vi "Stop.vi"(0 "object in":refnum<class "CetoniPump.lvclass">, 2 "index":i32, 5 "error in (no error)":errorcluster) -> (14 "object out":refnum<class "CetoniPump.lvclass">, 19 "error out":errorcluster)   [LabVIEW 2023, in "CetoniPump.lvclass"]
uses:
  CetoniPump.lvclass
  CetoniPump.lvclass/CetoniPump.ctl
  CETONI_SDK/lib/labview/labbCAN_Pump_API/labbCAN_Pump_API.lvlib
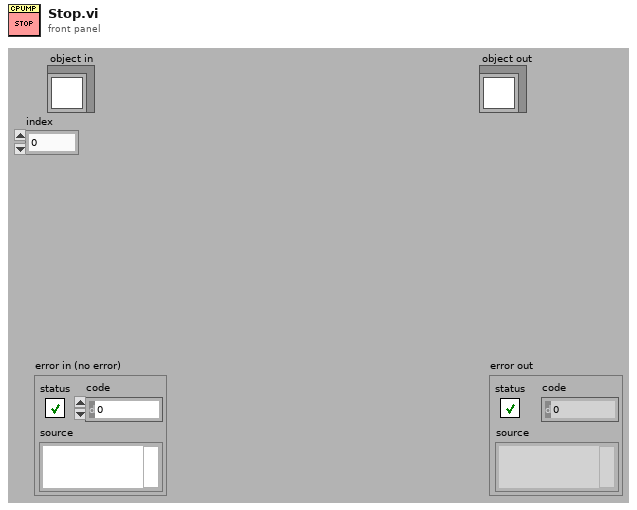
[diagram p1: front panel]
types:
  T1 = cluster{"Pump Handle":i64, "Pump Name":string, "Maximum Volume":dbl, "Maximum Flow Rate":dbl, "Flow Rate":dbl, "Target Level":dbl, "Valve Handle":i64, "Has Valve?":bool, "Actual valve position":i32}[]
  T2 = cluster{"Pump Handle":i64, "Pump Name":string, "Maximum Volume":dbl, "Maximum Flow Rate":dbl, "Flow Rate":dbl, "Target Level":dbl, "Valve Handle":i64, "Has Valve?":bool, "Actual valve position":i32}
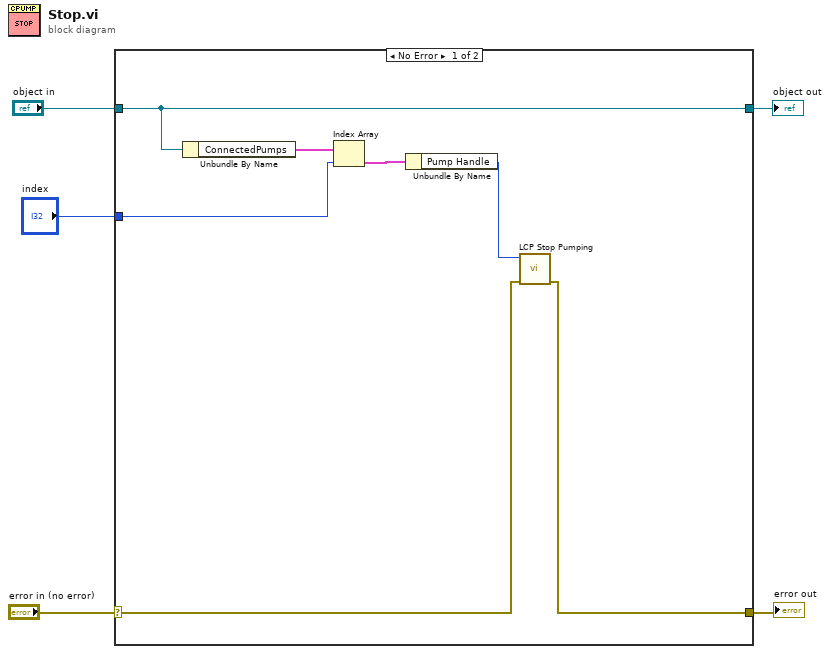
[diagram p0: block diagram]
diagram:
  n1 = case shown="No Error" "error in (no error)" {
    selector: "error in (no error)" -> [w11 w14]
    tunnel: [w10 w14] -> w4
    tunnel: [w12 w13] -> w2
    tunnel: "object in" -> [w12 w13]
    tunnel: "index" -> [w6 _]
    frame No Error {
      n2 = Unbundle By Name(w12) -> ("ConnectedPumps"=w8:T1)
      n3 = Index Array(array=w8, index=w6) -> (element=w9:T2)
      n4 = Unbundle By Name(w9) -> ("Pump Handle"=w7:i64)
      n5 = call "LCP Stop Pumping.vi"("error in (no error)"=w11, "Pump Handle"=w7) -> ("error out"=w10:errorcluster)  [unwired: 9 in]
    }
    frame Error {
    }
  }
  "error out" <- w4
  "object out" <- w2
